vi "MALTCON get value of miant counter.vi"() -> ()   [LabVIEW 2018]
uses:
  <instrlib>/AltonTech MALT/AltonTech MALT200817.lvlib
panel:
  in  "Address":i32=1
  out "Value":u32
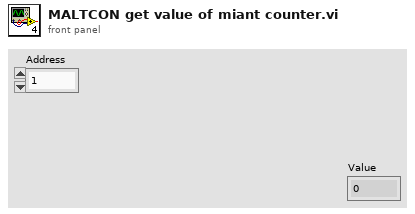
[diagram p1: front panel]
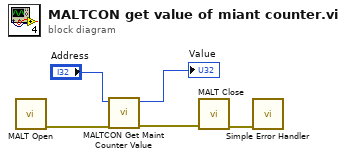
[diagram p0: block diagram]
diagram:
  n1 = call <instrlib>:"MALT Open.vi"() -> ("error out"=w3:errorcluster)  [unwired: 10 in, 1 out]
  n2 = call <instrlib>:"MALTCON Get Maint Counter Value.vi"("error in"=w3, "Address"="Address") -> ("error out"=w2:errorcluster, "Value"=→"Value":u32)  [unwired: 8 in]
  n3 = call <instrlib>:"MALT Close.vi"("error in"=w2) -> ("error out"=w5:errorcluster)  [unwired: 10 in]
  n4 = call <vilib>:"Simple Error Handler.vi"("error in (no error)"=w5) -> ()  [unwired: 4 in, 5 out]
